vi "Array - Insert on top.vi"(0 "New Array(1D)":string[](array[string]), 5 "Input Array(2D)":string[][](array[string])) -> (6 "Output Array(2D)":string[][](array[string]))   [LabVIEW 2009]
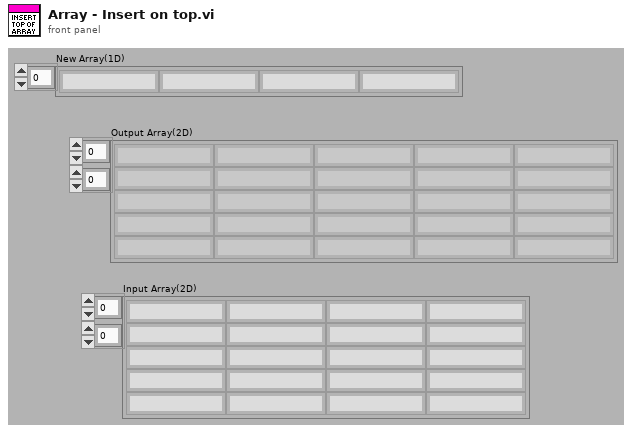
[diagram p1: front panel]
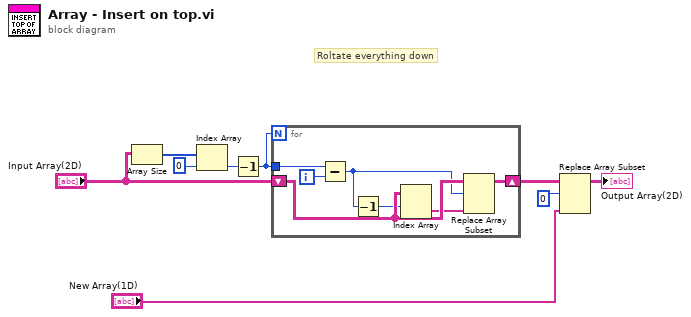
[diagram p0: block diagram]
diagram:
  # "Roltate everything down"
  n1 = Array Size(array="Input Array(2D)") -> (size(s)=w9:i32[])
  n2 = Index Array(array=w9, index=0) -> (element=w7:i32)
  n3 = Decrement(x=w7) -> (x-1=w6:i32)
  n4 = for {
    N: w6 -> [_]
    tunnel: w6 -> [w16]
    shift-right: [w11] -> w4
    shift-left: "Input Array(2D)" -> [w15]
    i -> [w12]
    n5 = Subtract(x=w16, y=w12) -> (x-y=w10:i32)
    n6 = Decrement(x=w10) -> (x-1=w13:i32)
    n7 = Index Array(array=w15, index (row)=w13) -> (element=w14:string[])  [unwired: 1 in]
    n8 = Replace Array Subset(array=w15, new element=w14, index (row)=w10) -> (w11:string[][])  [unwired: 1 in]
  }
  n9 = Replace Array Subset(array=w4, new element="New Array(1D)", index (row)=0) -> (→"Output Array(2D)":string[][])  [unwired: 1 in]
